vi "Create User Event - Stop.vi"(8 "error in (no error)":errorcluster) -> (0 "error out":errorcluster, 2 "User Event - Stop":refnum<user-event>, 3 "Event Registration Refnum Out":refnum<event-registration>)   [LabVIEW 2019, in "User Event - Stop.lvlib"]
doc: "Create a boolean user event that will be used to stop the event loop from the message handling loop."
uses:
  User Event - Stop.lvlib
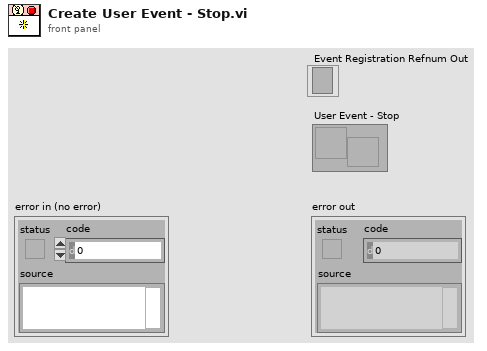
[diagram p1: front panel]
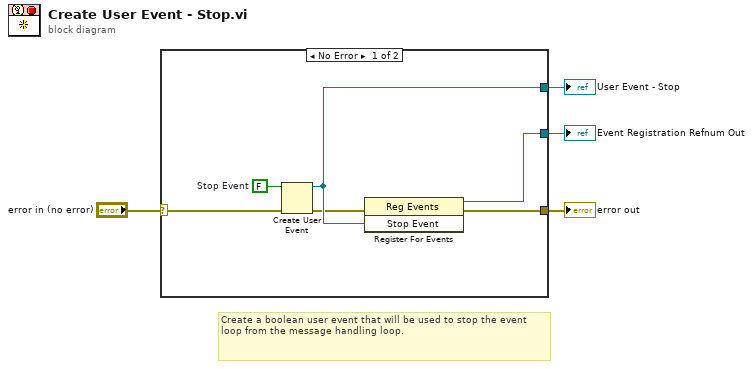
[diagram p0: block diagram]
diagram:
  # "Create a boolean user event that will be used to stop the event loop from the message handling loop."
  n1 = case shown="No Error" "error in (no error)" {
    selector: "error in (no error)" -> [w7 w11]
    tunnel: [w10 _] -> w4
    tunnel: [w6 _] -> w1
    tunnel: [w8 w11] -> w3
    frame No Error {
      w5 = FALSE  # Stop Event
      n2 = Create User Event(user event datatype=w5, error in=w7) -> (user event=w10:refnum<user-event>, error out=w9:errorcluster)
      n3 = register-events(error in=w9, w10) -> (reference out=w6:refnum<event-registration>, error out=w8:errorcluster)  [unwired: 1 in]
    }
    frame Error {
    }
  }
  "User Event - Stop" <- w4
  "error out" <- w3
  "Event Registration Refnum Out" <- w1
